vi "Reduce Fraction.vi"(4 "denominator":u16, 5 "numerator":u16) -> (1 "reduced denominator":u16, 2 "reduced numerator":u16)   [LabVIEW 2016]
doc: "This VI Takes two numbers and divides them by their Greatest Common Denominator. This gives us the ratio between the two values in the smallest integer form."
uses:
  <vilib>/gmath/NI_Gmath.lvlib
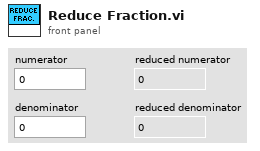
[diagram p1: front panel]
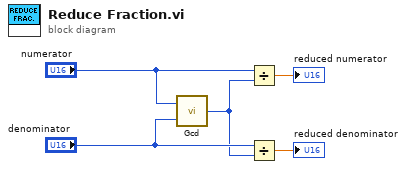
[diagram p0: block diagram]
diagram:
  n1 = call <vilib>:"Gcd.vi"("y"="denominator", "x"="numerator") -> ("gcd(x,y)"=w3:i32)
  n2 = Divide(x="numerator", y=w3) -> (x/y=→"reduced numerator":dbl)
  n3 = Divide(x="denominator", y=w3) -> (x/y=→"reduced denominator":dbl)
